vi "CheckAscriptIntegrity_DashSide.vi"(10 "UseUploadedPath?":bool, 11 "UploadedAscript":path) -> (2 "BotAscriptName":string, 3 "AscriptIntegrityGood?":bool)   [LabVIEW 2016]
uses:
  <vilib>/Rock Robotics/Network Tables/NT Read String.vi
  <vilib>/Rock Robotics/Network Tables/NT Read Boolean.vi
panel:
  in  "Base Path":path
  out "MatchingFileFound":bool
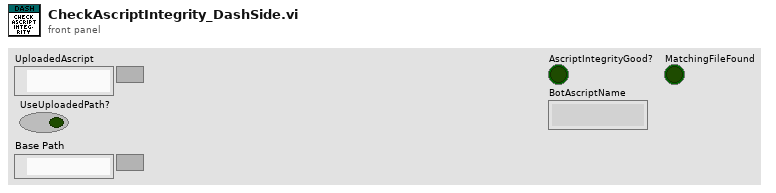
[diagram p1: front panel]
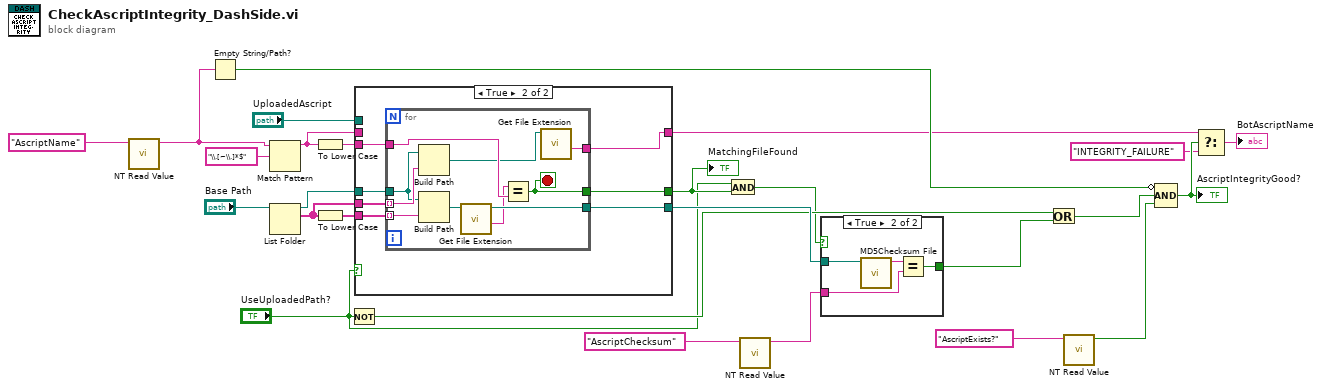
[diagram p0: block diagram]
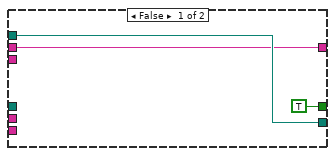
[diagram p2: hidden frame]
diagram:
  n1 = call-poly <vilib>:"NT Read Value.vi"("Name"="AscriptName") -> ("String"=w10:string)  [unwired: 9 in, 1 out]
  n2 = Empty String/Path?(string/path=w10) -> (empty?=w15:bool)
  n3 = Match Pattern(string=w10, regular expression="\\.[~\\.]*$") -> (before substring=w7:string)  [unwired: 4 out]
  n4 = List Folder(path="Base Path") -> (path out=w11:path, filenames=w5:string[])  [unwired: 3 in, 2 out]
  n5 = To Lower Case(string=w7) -> (all lower case string=w9:string)
  n6 = To Lower Case(string=w5) -> (all lower case string=w23:string[])
  n7 = Not(x="UseUploadedPath?") -> (.not. x?=w13:bool)
  n8 = case shown="True" "UseUploadedPath?" {
    tunnel: w23 -> [_ w36]
    tunnel: w9 -> [_ w35]
    tunnel: [w28 w34] -> w21
    tunnel: [TRUE w33] -> w4
    tunnel: [w27 w32] -> w6
    tunnel: w11 -> [_ w31]
    tunnel: "UploadedAscript" -> [w28 _]
    tunnel: w7 -> [w27 _]
    tunnel: w5 -> [_ w30]
    frame False {
    }
    frame True {
      n9 = for {
        tunnel: w36 -> [w42] mode=indexing
        tunnel: w31 -> [w37]
        tunnel: w35 -> [w45]
        tunnel: [w44] -> w33
        tunnel: [w43] -> w34
        tunnel: [w38] -> w32
        tunnel: w30 -> [w39] mode=indexing
        stop <- w44 stop-if-true
        n10 = Build Path(base path=w37, name or relative path=w39) -> (appended path=w40:path)
        n11 = Build Path(base path=w37, name or relative path=w42) -> (appended path=w46:path)
        n12 = call <vilib>:"Get File Extension.vi"("file"=w46) -> ("filename without extension"=w41:string, "dup file"=w43:path)  [unwired: 6 in, 3 out]
        n13 = Equal?(x=w41, y=w45) -> (x = y?=w44:bool)
        n14 = call <vilib>:"Get File Extension.vi"("file"=w40) -> ("filename without extension"=w38:string)  [unwired: 6 in, 4 out]
      }
    }
  }
  "MatchingFileFound" <- w4
  n15 = And(x="UseUploadedPath?", y=w4) -> (x .and. y?=w3:bool)
  n16 = call-poly <vilib>:"NT Read Value.vi"("Name"="AscriptChecksum") -> ("String"=w20:string)  [unwired: 9 in, 1 out]
  n17 = case shown="True" w3 {
    tunnel: w21 -> [_ w50]
    tunnel: w20 -> [_ w48]
    tunnel: [_ w47] -> w14
    frame False {
    }
    frame True {
      n18 = call <vilib>:"MD5Checksum File.vi"("Path"=w50) -> ("MD5 message-digest"=w49:string)  [unwired: 9 in, 1 out]
      n19 = Equal?(x=w49, y=w48) -> (x = y?=w47:bool)
    }
  }
  n20 = Or(x=w13, y=w14) -> (x .or. y?=w12:bool)
  n21 = call-poly <vilib>:"NT Read Value.vi"("Name"="AscriptExists?") -> ("Boolean"=w19:bool)  [unwired: 9 in, 1 out]
  n22 = Compound Arithmetic op=AND(invert w15, w12, w19) -> (w18:bool)
  "AscriptIntegrityGood?" <- w18
  n23 = Select(t=w6, s=w18, f="INTEGRITY_FAILURE") -> (s? t:f=→"BotAscriptName":string)
